vi "Handling.vi"   [LabVIEW 2015]
uses:
  Vision/Vision Published Globals.vi
  Intake/Implementation/Intake Published Globals.vi
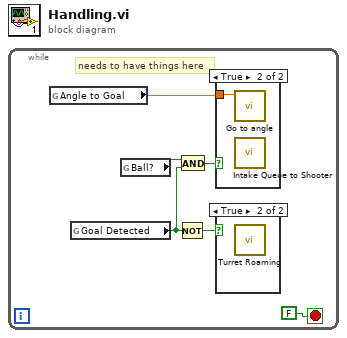
[diagram p0: block diagram]
diagram:
  n1 = while {
    stop <- FALSE stop-if-true
    # "needs to have things here"
    n2 = global read "Vision Published Globals.vi" "Angle to Goal"() -> (w4:dbl)
    n3 = global read "Vision Published Globals.vi" "Goal Detected"() -> (w2:bool)
    n4 = global read "Intake Published Globals.vi" "Ball?"() -> (w3:bool)
    n5 = Not(x=w2) -> (.not. x?=w1:bool)
    n6 = And(x=w3, y=w2) -> (x .and. y?=w6:bool)
    n7 = case shown="True" w6 {
      tunnel: w4 -> [_ w7]
      frame False {
      }
      frame True {
        n8 = call "Go to angle.vi"("Setpoint"=w7) -> ()  [unwired: 10 in, 1 out]
        n9 = call "Intake Queue to Shooter.vi"() -> ()  [unwired: 11 in, 1 out]
      }
    }
    n10 = case shown="True" w1 {
      frame False {
      }
      frame True {
        n11 = call "Turret Roaming.vi"() -> ()  [unwired: 11 in, 1 out]
      }
    }
  }
